vi "nD Nonlinear System Solver.vi"   [LabVIEW 2010, in "NI_Gmath.lvlib"]
doc: "Determines a set of solutions of a nonlinear system of equations in n dimensions beginning with a randomly chosen start point in n dimensions. You must manually select the polymorphic instance to use."
uses:
  NI_Gmath.lvlib
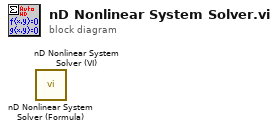
[diagram p0: block diagram]
diagram:
  n1 = call "nD Nonlinear System Solver (Formula).vi"() -> ()  [unwired: 8 in, 4 out]
  n2 = call "nD Nonlinear System Solver (VI).vi"() -> ()  [unwired: 8 in, 4 out]
